vi "Read Next Msg.vi"(8 "error in":errorcluster, 9 "Termination (Exit)":string="Exit", 10 "timeout (-1ms)":i32=-1, 11 "Msg Queue In":refnum<queue>) -> (0 "error out":errorcluster, 1 "Msg Value":variant, 2 "Msg Name":string, 3 "Msg Queue Out":refnum<queue>, 4 "Stop?":bool, 5 "timed out?":bool, 6 "Q Backlog":i32)   [LabVIEW 2018, in "EZ Message.lvlib"]
uses:
  EZ Message.lvlib
  Message.ctl
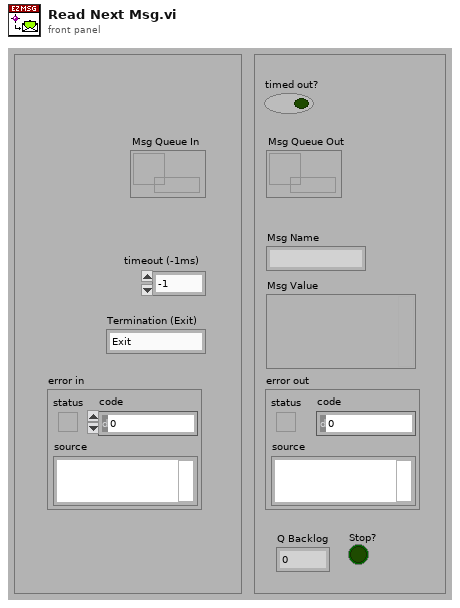
[diagram p1: front panel]
types:
  T1 = typedef "EZ Message.lvlib/Message.ctl" = cluster{"Name":string, "Value":variant}
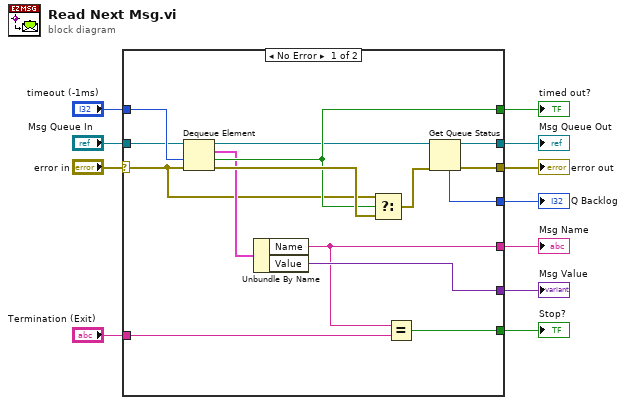
[diagram p0: block diagram]
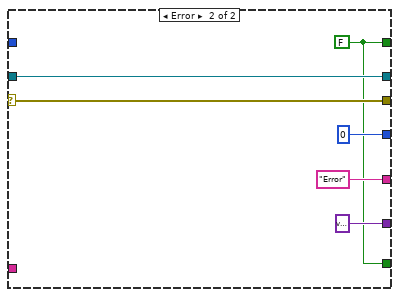
[diagram p2: hidden frame]
diagram:
  n1 = case shown="No Error" "error in" {
    selector: "error in" -> [w15 w32]
    tunnel: [w13 "Error" ("Name")] -> w11
    tunnel: [w24 w27] -> w10
    tunnel: [w23 w31] -> w9
    tunnel: [w22 w32] -> w8
    tunnel: [w21 variant ("Value")] -> w7
    tunnel: [w20 0 ("# elements in queue")] -> w6
    tunnel: "timeout (-1ms)" -> [w18 _]
    tunnel: "Msg Queue In" -> [w17 w31]
    tunnel: "Termination (Exit)" -> [w14 _]
    tunnel: [w12 w27] -> w1
    frame No Error {
      n2 = Dequeue Element(queue=w17, timeout in ms (-1)=w18, error in (no error)=w15) -> (queue out=w16:refnum<queue>, element=w19:T1, timed out?=w24:bool, error out=w25:errorcluster)
      n3 = Unbundle By Name(w19) -> ("Name"=w13:string, "Value"=w21:variant)
      n4 = Select(t=w15, s=w24, f=w25) -> (s? t:f=w26:errorcluster)
      n5 = Equal?(x=w13, y=w14) -> (x = y?=w12:bool)
      n6 = Get Queue Status(queue=w16, error in (no error)=w26) -> (queue out=w23:refnum<queue>, error out=w22:errorcluster, # elements in queue=w20:i32)  [unwired: 1 in, 5 out]
    }
    frame Error {
      w27 = FALSE ("timed out?")
    }
  }
  "Msg Name" <- w11
  "timed out?" <- w10
  "Msg Queue Out" <- w9
  "error out" <- w8
  "Msg Value" <- w7
  "Q Backlog" <- w6
  "Stop?" <- w1
